vi "prediction_loop.vi"(8 "error in":errorcluster) -> (0 "error out":errorcluster)   [LabVIEW 2010]
uses:
  <vilib>/Platform/TimedLoop/XDataNode/XDataNode.xnode
  <vilib>/Platform/TimedLoop/XDataNode/timing_clust.ctl
  <vilib>/Platform/TimedLoop/XDataNode/nitl_modes.ctl
  <vilib>/Platform/TimedLoop/XDataNode/wakeup.ctl
  initialization/micron_globals.vi
  <vilib>/Platform/TimedLoop/XDataNode/XDNodeRunTimeDep.lvlib
panel:
  in  "u0":dbl=1.67e-05
  in  "u":dbl=0.0167
  out "Prediction Lookahead":sgl
  in  "FFT Length":i32=128
  in  "Sampling frequency":sgl=1000.0
  # "Locals:"
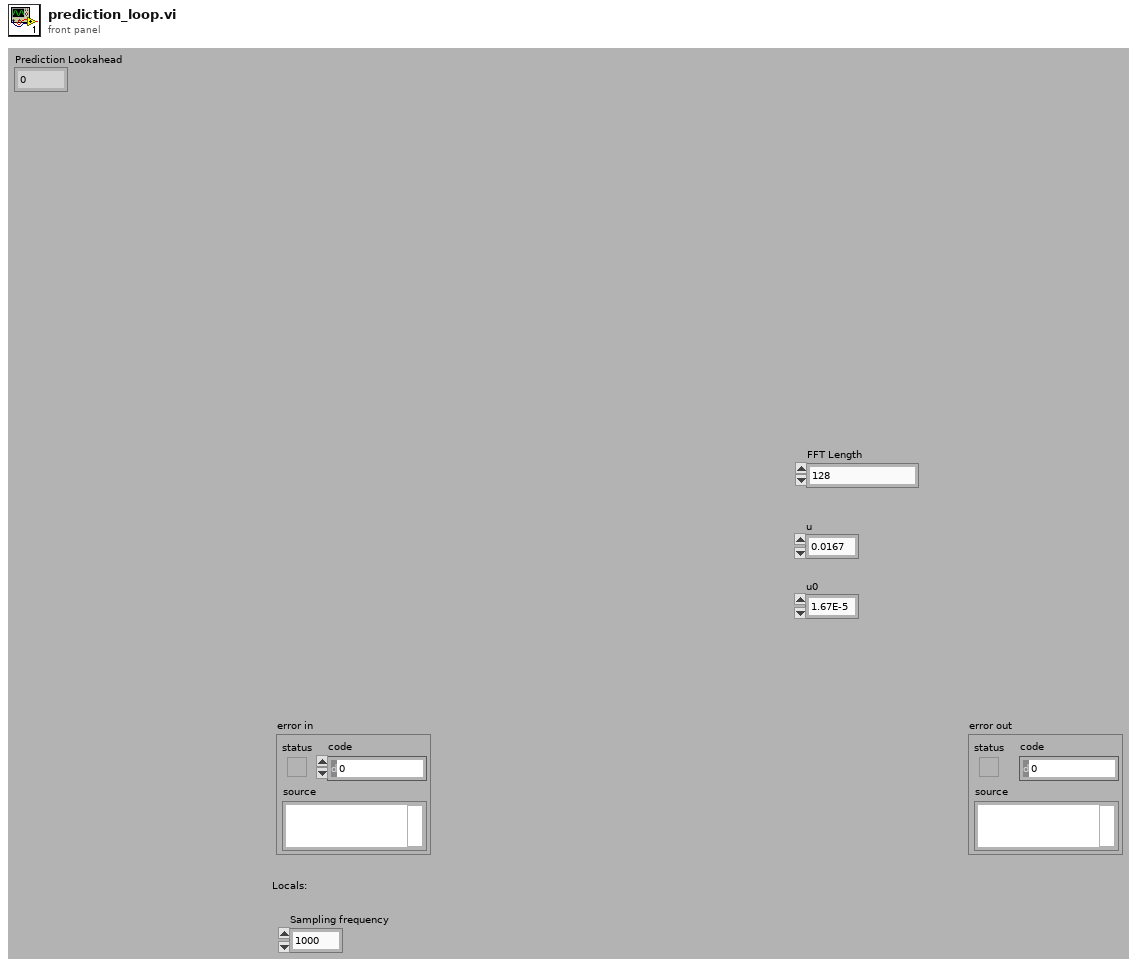
[diagram p1: front panel]
types:
  T1 = typedef "Micron params.ctl" = cluster{"Stimulus":T2, "Goal Filter A":T4, "Mode controls":T5, "Manipulator type":enum16{"Current piezo", "Voltage piezo"}, "Manipulator calibration":T6, "Network":T8, "Goal Filter B":T4, "Cancellation":T9, "Transition time":sgl, "Estimation and Feedforward":cluster{"Use Raw Data (ignore Kalman Filter)":bool, "Turn Kalman Filter Off":bool, "Use IMC (if off, PID is used)":bool, "KP":sgl, "KI":sgl, "KD":sgl, "Feedforward Control":bool, "Velocity Gain":dbl[], "KF input delay":i32}}
  T2 = typedef "stimulus.ctl" = cluster{"Type":enum16{"Off", "Step", "Sine", "Triangle", "Arbitrary"}, "Delay":i32, "Amplitude":sgl[], "Injection point":T3, "Closed loop":bool, "Offset":sgl[], "Tip -> world":bool}
  T3 = typedef "injection_point.ctl" = enum16{"Total pose", "V limiter", "Goal ", "Link position", "Link rate", "Link residue", "Link goal", "Link error", "Controller", "Output", "DAC"}
  T4 = typedef "goal_filter_parms.ctl" = cluster{"Lower Fc":sgl, "Lower Q":sgl, "Scale factor":sgl, "Upper Fc":sgl, "Upper Q":sgl, "Manip zeroing":sgl, "Speedup max":sgl, "Speedup thresh":sgl, "Speedup nonlin":sgl, "V limit":sgl, "V limit range":sgl}
  T5 = typedef "mode_conrols.ctl" = cluster{"Hold":bool, "Cancellation":bool, "Goal filter":bool, "Trigger":bool}
  T6 = typedef "manipulator_cal.ctl" = cluster{"Tip offset":sgl[], "Tip light calibration":T7, "Axial filter":cluster{"filter structure":enum32{"IIR 2nd Order", "IIR 4th Order"}, "Reverse Coefficients":dbl[], "Forward Coefficients":dbl[]}, "Lateral filter":cluster{"filter structure":enum32{"IIR 2nd Order", "IIR 4th Order"}, "Reverse Coefficients":dbl[], "Forward Coefficients":dbl[]}, "Handle light calibration":T7, "RCM offset":sgl[], "Base pivots":sgl[][], "Output pivots":sgl[][], "Length center":sgl}
  T7 = typedef "probe_calibration.ctl" = sgl[][]
  T8 = typedef "network_params.ctl" = cluster{"Remote Host":string, "Send Status":bool, "Send Port":u16, "Recv Commands":bool, "Recv Port":u16}
  T9 = typedef "im_control_params.ctl" = cluster{"Bandwidth":sgl, "Delay":i32, "Stack travel":sgl, "Saturation pos":sgl, "Slew Limit":sgl, "Turnoff zeroing":sgl, "Bypass":bool}
  T10 = typedef "XDNodeRunTimeDep.lvlib/timing_clust.ctl" = cluster{"Expected End [f-1]":u64, "Actual End [f-1]":u64, "Finished Late? [f-1]":bool, "Expected End [i-1]":u64, "Actual End [i-1]":u64, "Finished Late? [i-1]":bool, "Expected Start [i]":u64, "Actual Start [i]":u64, "Expected Start [f]":u64, "Actual Start [f]":u64, "Source Name":string, "Structure Name":string, "Period":i64, "Deadline":i64, "Offset":i64, "Start":i64, "Priority":i32, "Timeout":i32, "Mode":T11, "Wakeup Reason":T12, "Error":errorcluster, "Source Type":string, "Secondary Source Type":string, "Global End Time":u64, "Global Start Time":u64, "Frame Duration":u64, "Iteration Duration":u64, "Assigned CPU":i32, "I/O Scan Engine Mode":u32}
  T11 = typedef "XDNodeRunTimeDep.lvlib/nitl_modes.ctl" = enum32{"No Change", "Process missed periods, maintain original phase", "Discard missed periods, maintain original phase", "Process missed periods, ignore original phase", "Discard missed periods, ignore original phase"}
  T12 = typedef "XDNodeRunTimeDep.lvlib/wakeup.ctl" = enum32{"Normal", "Aborted", "Asynchronous wakeup", "Timing source error", "Timed loop error", "Timeout"}
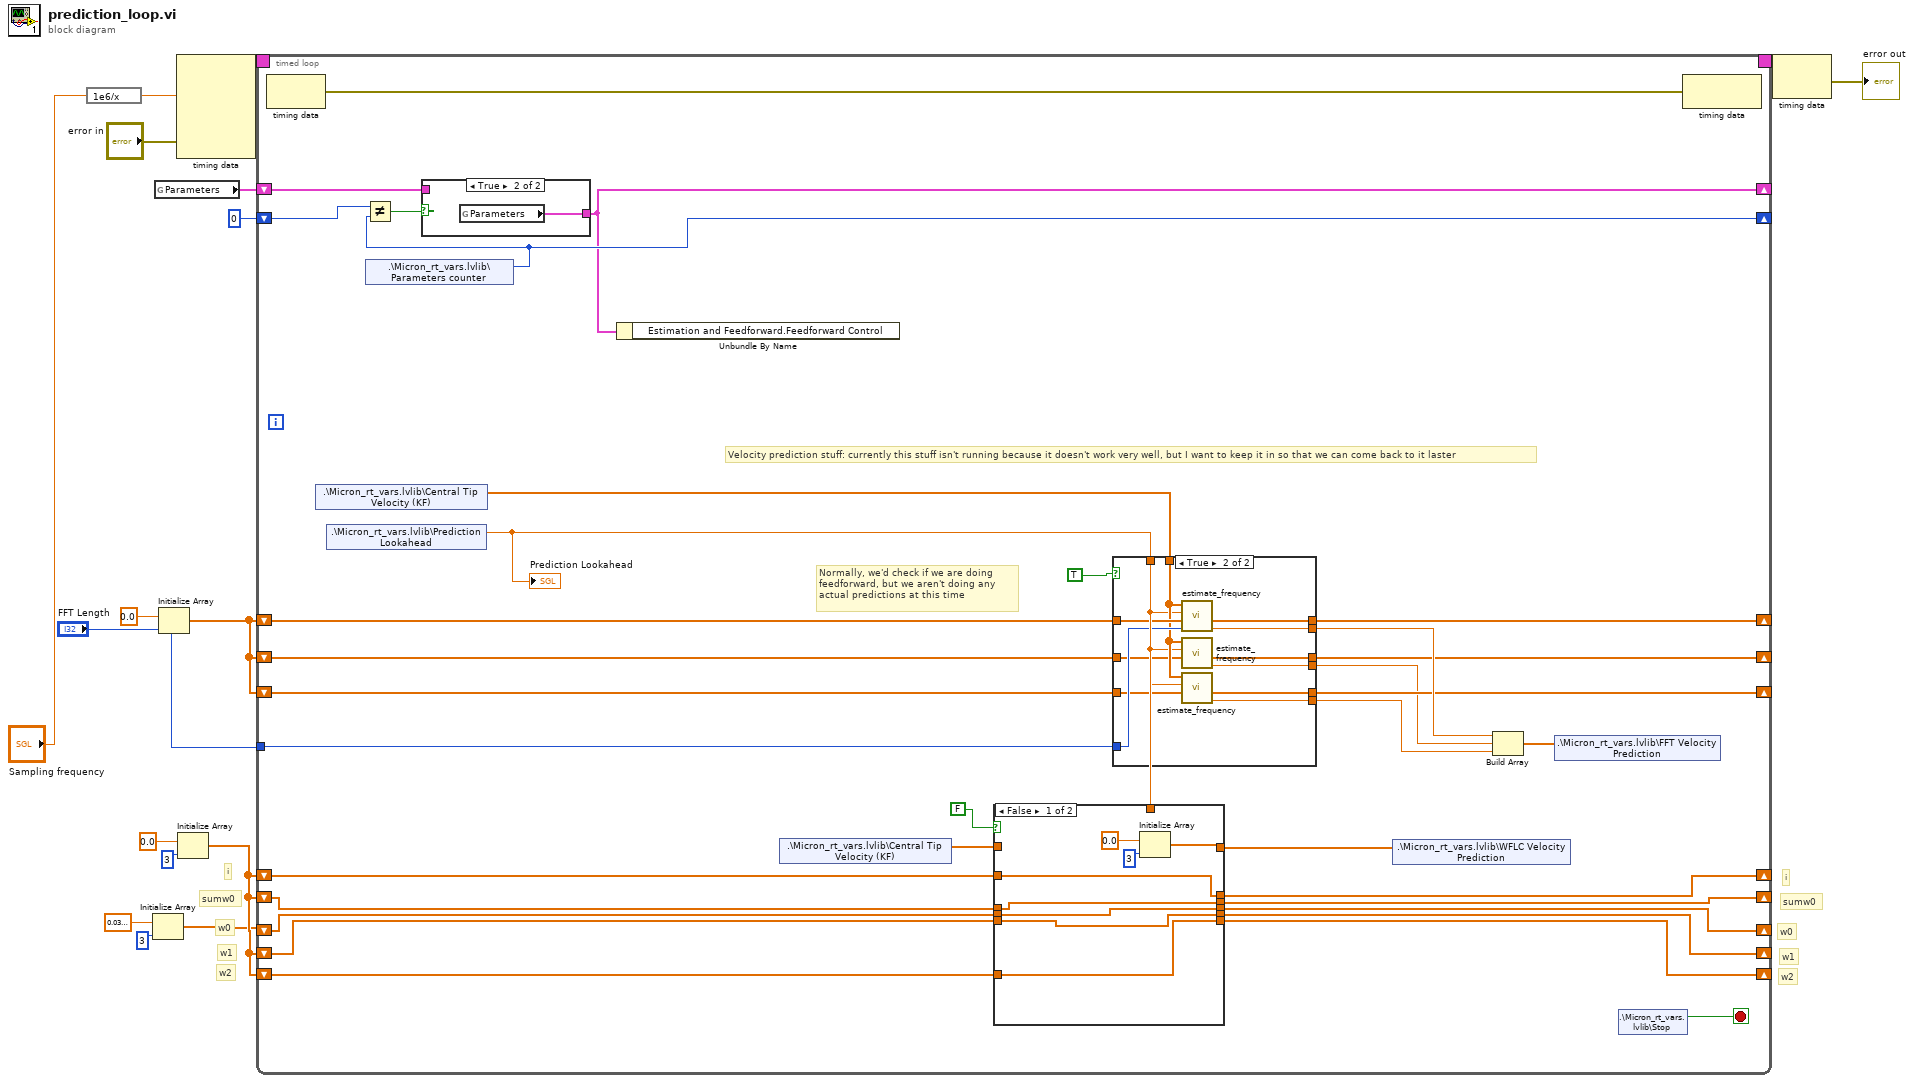
[diagram p0: block diagram]
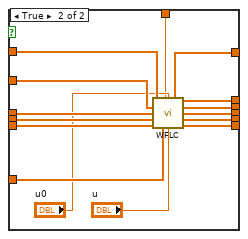
[diagram p2: hidden frame]
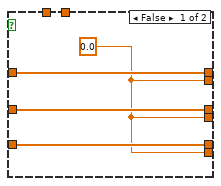
[diagram p3: hidden frame]
diagram:
  # "sumw0"
  # "i"
  # "w1"
  # "w2"
  # "w0"
  # "sumw0"
  # "i"
  # "w1"
  # "w2"
  # "w0"
  n1 = expression code="1e6/x"("Sampling frequency") -> (w12:sgl)
  n2 = Initialize Array(sgl 0.04 ("t"), 3 ("t")) -> (w2:sgl[])
  n3 = global read "micron_globals.vi" "Parameters"() -> (w10:T1)
  n4 = Initialize Array(sgl 0.0 ("t"), "FFT Length") -> (w1:sgl[])
  n5 = node-c288(w12, "error in") -> (w17:T10)  [unwired: 3 out]
  n6 = Initialize Array(sgl 0.0 ("t"), 3 ("t")) -> (w5:sgl[])
  n7 = timed-loop {
    timing: w17 -> [_]
    timing-out: [_] -> w16
    shift-right: [w18] -> _
    shift-left: w10 -> [w46]
    shift-right: [w47] -> _
    shift-left: u32 0 ("Parameters counter") -> [w48]
    shift-right: [w43] -> _
    shift-left: w1 -> [w45]
    tunnel: "FFT Length" -> [w44]
    shift-right: [w34] -> _
    shift-left: w2 -> [w36]
    shift-right: [w31] -> _
    shift-left: w5 -> [w32]
    shift-right: [w30] -> _
    shift-left: w5 -> [w33]
    shift-right: [w40] -> _
    shift-left: w5 -> [w38]
    shift-right: [w35] -> _
    shift-left: w5 -> [w39]
    shift-right: [w25] -> _
    shift-left: w1 -> [w27]
    shift-right: [w24] -> _
    shift-left: w1 -> [w26]
    stop <- w50 stop-if-true
    # "Normally, we'd check if we are doing \nfeedforward, but we aren't doing any\nactual predictions at this time"
    # "Velocity prediction stuff: currently this stuff isn't running because it doesn't work very well, but I want to keep it in so that we can come back to it laster"
    n8 = node-c288() -> (w51:errorcluster)  [unwired: 1 out]
    n9 = shared-variable ".\\Micron_rt_vars.lvlib\\Central Tip Velocity (KF)"() -> (w28:sgl[])  [unwired: 2 out]
    n10 = shared-variable ".\\Micron_rt_vars.lvlib\\Prediction Lookahead"() -> (w21:sgl)  [unwired: 1 in, 1 out]
    "Prediction Lookahead" <- w21
    n11 = shared-variable ".\\Micron_rt_vars.lvlib\\Parameters counter"() -> (w47:u32)  [unwired: 2 out]
    n12 = Not Equal?(x=w48, y=w47) -> (x != y?=w49:bool)
    n13 = case shown="True" w49 {
      tunnel: [w91 w92] -> w18
      tunnel: w46 -> [w91 _]
      frame False {
      }
      frame True {
        n14 = global read "micron_globals.vi" "Parameters"() -> (w92:T1)
      }
    }
    n15 = Unbundle By Name(w18) -> ()  [unwired: 1 out]
    n16 = shared-variable ".\\Micron_rt_vars.lvlib\\Central Tip Velocity (KF)"() -> (w37:sgl[])  [unwired: 2 out]
    n17 = case shown="False" FALSE {
      tunnel: [w59 w74] -> w40
      tunnel: w39 -> [w58 w73]
      tunnel: w38 -> [w59 w72]
      tunnel: w37 -> [_ w71]
      tunnel: w36 -> [w57 w70]
      tunnel: [w58 w69] -> w35
      tunnel: [w57 w68] -> w34
      tunnel: w33 -> [w56 w67]
      tunnel: w32 -> [w55 w66]
      tunnel: [w55 w65] -> w31
      tunnel: [w56 w64] -> w30
      tunnel: [w52 w63] -> w29
      tunnel: w21 -> [_ w60]
      frame False {
        n18 = Initialize Array(sgl 0.0 ("t"), 3 ("t")) -> (w52:sgl[])
      }
      frame True {
        n19 = call "WFLC.vi"("Prediction Lookahead"=w60, "Signal"=w71, "u0"="u0", "i"=w72, "sumw0"=w73, "w0"=w70, "w1"=w66, "w2"=w67, "u"="u") -> ("out i"=w74:sgl[], "out sumw0"=w69:dbl[], "out w0"=w68:dbl[], "out w1"=w65:dbl[], "Prediction"=w63:dbl[], "out w2"=w64:dbl[])  [unwired: 1 in]
      }
    }
    n20 = case shown="True" TRUE {
      tunnel: w45 -> [w78 w90]
      tunnel: w44 -> [_ w89]
      tunnel: [w78 w88] -> w43
      tunnel: [w75 w87] -> w41
      tunnel: w28 -> [_ w86]
      tunnel: w27 -> [w77 w85]
      tunnel: w26 -> [w76 w84]
      tunnel: [w77 w83] -> w25
      tunnel: [w76 w82] -> w24
      tunnel: [w75 w81] -> w23
      tunnel: [w75 w80] -> w22
      tunnel: w21 -> [_ w79]
      frame False {
        w75 = sgl 0.0 ("t")
      }
      frame True {
        n21 = call "estimate_frequency.vi"("FFT Length"=w89, "State In"=w90, "Prediction Lookahead"=w79, "Central Tip Position (KF)"=w86) -> ("Prediction"=w87:dbl, "State Out"=w88:sgl[])  [unwired: 2 out]
        n22 = call "estimate_frequency.vi"("State In"=w85, "Prediction Lookahead"=w79, "Central Tip Position (KF)"=w86) -> ("Prediction"=w81:dbl, "State Out"=w83:sgl[])  [unwired: 1 in, 2 out]
        n23 = call "estimate_frequency.vi"("State In"=w84, "Prediction Lookahead"=w79, "Central Tip Position (KF)"=w86) -> ("Prediction"=w80:dbl, "State Out"=w82:sgl[])  [unwired: 1 in, 2 out]
      }
    }
    n24 = shared-variable ".\\Micron_rt_vars.lvlib\\WFLC Velocity Prediction"(w29) -> ()  [unwired: 1 in, 1 out]
    n25 = Build Array(w41, w23, w22) -> (w42:dbl[])
    n26 = shared-variable ".\\Micron_rt_vars.lvlib\\FFT Velocity Prediction"(w42) -> ()  [unwired: 1 in, 1 out]
    n27 = shared-variable ".\\Micron_rt_vars.lvlib\\Stop"() -> (w50:bool)  [unwired: 2 out]
    n28 = node-c288(w51) -> ()  [unwired: 1 out]
  }
  n29 = node-c288(w16) -> (→"error out":errorcluster)
